vi "Buttons Latching Read.vi"(4 "error in (no error)":errorcluster, 6 "Container State":T3, 7 "Display State In":T1={"Buttons Displayed"=0, "Button States"=[], "Button Size"=0, "Button Style"=enum."Classic", "Active Button"=0, "Force Regen?"=FALSE, "Tip String Ref"=refnum}) -> (0 "error out":errorcluster, 2 "Value":bool[](array[boolean]), 3 "Display State Out":T1={"Buttons Displayed"=0, "Button States"=[], "Button Size"=0, "Button Style"=enum."Classic", "Active Button"=0, "Force Regen?"=FALSE, "Tip String Ref"=refnum})   [LabVIEW 2012, in "Toolbar.xctl"]
doc: "Read which of the toolbar buttons are latching type buttons"
uses:
  Toolbar.xctl
  <vilib>/_xctls/Container State.ctl
  Toolbar State.ctl
  Button_Class/Button.lvclass
  Button_Class/Type Defs/Button Style.ctl
  Button_Class/Type Defs/Button Type.ctl
  <vilib>/_xctls/XControlSupport.lvlib
panel:
  # "Replace the Value Indicator below with an Indicator of desired type.\nDo not remove this Indicator or the others from the connector pane. \nDo not change the connector pane pattern.\nThe Value Indicator should always be the second terminal from top on the output side in the connector pane."
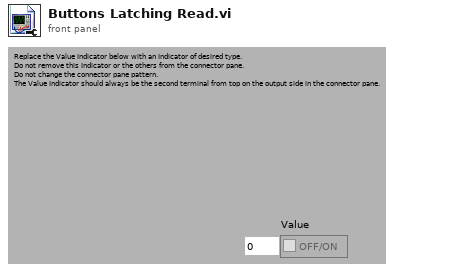
[diagram p1: front panel]
types:
  T1 = typedef "Toolbar.xctl/Toolbar State.ctl" = cluster{"Buttons Displayed":i32, "Button States":refnum<class "Button.lvclass">[], "Button Size":i32, "Button Style":T2, "Active Button":i32, "Force Regen?":bool, "Tip String Ref":refnum<vi>}
  T2 = typedef "Button.lvclass/Button Style.ctl" = enum16{"System", "Modern", "Classic", "Rounded", "Silver", "Ni Theme", "Metallic"}
  T3 = typedef "XControlSupport.lvlib/Container State.ctl" = cluster{"Indicator?":bool, "Run Mode?":bool, " Refnum":refnum<vi>}
  T4 = typedef "Button.lvclass/Button Type.ctl" = enum16{"Transitory", "Latching"}
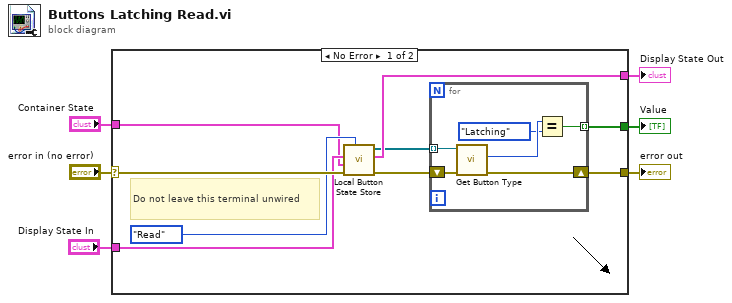
[diagram p0: block diagram]
diagram:
  n1 = case shown="No Error" "error in (no error)" {
    selector: "error in (no error)" -> [w12 w23]
    tunnel: [w15 _] -> w6
    tunnel: [w14 w23] -> w5
    tunnel: "Display State In" -> [w10 w22]
    tunnel: [w9 w22] -> w2
    tunnel: "Container State" -> [w8 _]
    frame No Error {
      # "Do not leave this terminal unwired"
      n2 = call "Local Button State Store.vi"("Operation"=enum16{"Read", "Write"}."Read", "error in (no error)"=w12, "Container State"=w8, "Display State In"=w10) -> ("error out"=w13:errorcluster, "Display State Out"=w9:T1, "Button States"=w7:refnum<class "Button.lvclass">[])  [unwired: 5 out]
      n3 = for {
        tunnel: w7 -> [w20] mode=indexing
        tunnel: [w21] -> w15 mode=indexing
        shift-right: [w17] -> w14
        shift-left: w13 -> [w18]
        n4 = call-dynamic "Get Button Type.vi"("error in (no error)"=w18, "Button in"=w20) -> ("error out"=w17:errorcluster, "Type"=w19:T4)  [unwired: 8 out]
        n5 = Equal?(x=w19, y=Button_Type."Latching") -> (x = y?=w21:bool)
      }
    }
    frame Error {
    }
  }
  "error out" <- w5
  "Display State Out" <- w2
  "Value" <- w6
